vi "Path Get From Ini.vi"(11 "Ini Path":path caption="配置文件的路径") -> (0 "电压/流-1":cluster{"电压（V）":dbl, "电流（A）":dbl}, 1 "扫条码？":bool, 2 "图片路径":path, 3 "配置文件路径":path, 4 "打印？":bool caption="打印", 5 "取反":bool[](array[boolean]), 6 "MES路径":path, 7 "测试台类型":string, 8 "测连锡":bool)   [LabVIEW 2011]
uses:
  <vilib>/Utility/config.llb/Read Key (String).vi
  <vilib>/Utility/config.llb/Read Key (Boolean).vi
  <vilib>/Utility/config.llb/Read Key (Double).vi
  <vilib>/Utility/config.llb/Write Key (Double).vi
  <vilib>/Utility/config.llb/Write Key (Boolean).vi
  <vilib>/Utility/config.llb/NI_LVConfig.lvlib
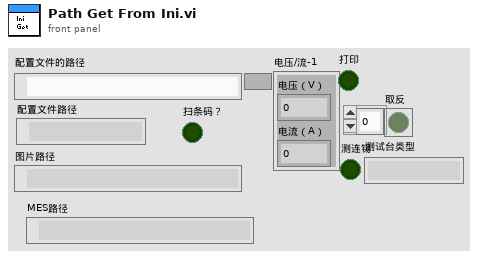
[diagram p1: front panel]
types:
  T1 = typedef "NI_LVConfig.lvlib/Config Data RefNum.ctl" = refnum<k1>
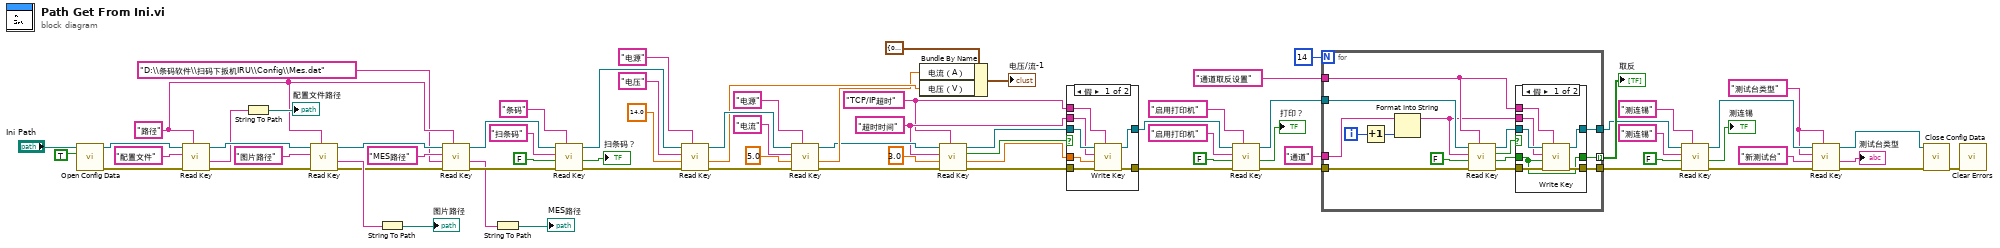
[diagram p0: block diagram]
diagram:
  w4 = "超时时间" ("key")
  w2 = "TCP/IP超时" ("section")
  w13 = "测试台类型" ("section")
  w35 = "路径" ("section")
  n1 = call <vilib>:"Open Config Data.vi"("create file if necessary (T)"=TRUE, "configuration file path"="Ini Path") -> ("error out"=w68:errorcluster, "refnum"=w74:T1)  [unwired: 7 in, 1 out]
  n2 = call-poly <vilib>:"Read Key.vi"("section"=w35, "error in (no error)"=w68, "key"="配置文件", "refnum"=w74) -> ("error out"=w67:errorcluster, "value"=w66:string, "refnum out"=w70:T1)  [unwired: 4 in, 1 out]
  n3 = String To Path(string=w66) -> (path=→"配置文件路径":path)
  n4 = call-poly <vilib>:"Read Key.vi"("section"=w35, "error in (no error)"=w67, "key"="图片路径", "refnum"=w70) -> ("error out"=w37:errorcluster, "value"=w65:string, "refnum out"=w39:T1)  [unwired: 4 in, 1 out]
  n5 = String To Path(string=w65) -> (path=→"图片路径":path)
  n6 = call-poly <vilib>:"Read Key.vi"("section"=w35, "error in (no error)"=w37, "default value"="D:\\条码软件\\扫码下扳机IRU\\Config\\Mes.dat", "key"="MES路径", "refnum"=w39) -> ("error out"=w36:errorcluster, "value"=w31:string, "refnum out"=w38:T1)  [unwired: 3 in, 1 out]
  n7 = String To Path(string=w31) -> (path=→"MES路径":path)
  n8 = call-poly <vilib>:"Read Key.vi"("section"="条码", "error in (no error)"=w36, "default value"=FALSE, "key"="扫条码", "refnum"=w38) -> ("error out"=w56:errorcluster, "value"=→"扫条码？":bool, "refnum out"=w57:T1)  [unwired: 3 in, 1 out]
  n9 = call-poly <vilib>:"Read Key.vi"("section"="电源", "error in (no error)"=w56, "default value"=14.0, "key"="电压", "refnum"=w57) -> ("error out"=w48:errorcluster, "value"=w45:dbl, "refnum out"=w49:T1)  [unwired: 3 in, 1 out]
  n10 = call-poly <vilib>:"Read Key.vi"("section"="电源", "error in (no error)"=w48, "default value"=5.0, "key"="电流", "refnum"=w49) -> ("error out"=w9:errorcluster, "value"=w44:dbl, "refnum out"=w10:T1)  [unwired: 3 in, 1 out]
  n11 = Bundle By Name(cluster=cluster{"电压（V）":dbl, "电流（A）":dbl} {"电压（V）"=0.0, "电流（A）"=0.0} ("电压/流-1 2"), "电流（A）"=w44, "电压（V）"=w45) -> (→"电压/流-1":cluster{"电压（V）":dbl, "电流（A）":dbl})
  n12 = call-poly <vilib>:"Read Key.vi"("section"=w2, "error in (no error)"=w9, "default value"=3.0, "key"=w4, "refnum"=w10) -> ("error out"=w7:errorcluster, "value"=w1:dbl, "found?"=w3:bool, "refnum out"=w8:T1)  [unwired: 3 in]
  n13 = case shown="假" w3 {
    tunnel: w8 -> [w81 w83]
    tunnel: w2 -> [w80 _]
    tunnel: w4 -> [w79 _]
    tunnel: w7 -> [w78 w82]
    tunnel: [w77 w82] -> w6
    tunnel: [w76 w83] -> w5
    tunnel: w1 -> [w75 _]
    frame False {
      n14 = call-poly <vilib>:"Write Key.vi"("section"=w80, "error in (no error)"=w78, "value"=w75, "key"=w79, "refnum"=w81) -> ("error out"=w77:errorcluster, "refnum out"=w76:T1)  [unwired: 4 in, 1 out]
    }
    frame True {
    }
  }
  n15 = call-poly <vilib>:"Read Key.vi"("section"="启用打印机", "error in (no error)"=w6, "default value"=FALSE, "key"="启用打印机", "refnum"=w5) -> ("error out"=w26:errorcluster, "value"=→"打印？":bool, "refnum out"=w27:T1)  [unwired: 3 in, 1 out]
  n16 = for {
    N: 14 -> [_]
    tunnel: w27 -> [w98]
    tunnel: w26 -> [w97]
    tunnel: "通道取反设置" ("名称或相对路径") -> [w90]
    tunnel: "通道" ("名称或相对路径") -> [w94]
    tunnel: [w87] -> w20
    tunnel: [w84] -> w21
    tunnel: [w86] -> w25 mode=indexing
    i -> [w96]
    n17 = Increment(x=w96) -> (x+1=w95:i32)
    n18 = Format Into String(initial string=w94, w95) -> (resulting string=w89:string)  [unwired: 2 in, 1 out]
    n19 = call-poly <vilib>:"Read Key.vi"("section"=w90, "error in (no error)"=w97, "default value"=FALSE, "key"=w89, "refnum"=w98) -> ("error out"=w88:errorcluster, "value"=w85:bool, "found?"=w92:bool, "refnum out"=w91:T1)  [unwired: 3 in]
    n20 = case shown="假" w92 {
      tunnel: w91 -> [w105 w108]
      tunnel: w90 -> [w104 _]
      tunnel: w89 -> [w103 _]
      tunnel: w88 -> [w102 w107]
      tunnel: [w101 w107] -> w87
      tunnel: [w100 w108] -> w84
      tunnel: [w99 w106] -> w86
      tunnel: w85 -> [w99 w106]
      frame False {
        n21 = call-poly <vilib>:"Write Key.vi"("section"=w104, "error in (no error)"=w102, "value"=w99, "key"=w103, "refnum"=w105) -> ("error out"=w101:errorcluster, "refnum out"=w100:T1)  [unwired: 4 in, 1 out]
      }
      frame True {
      }
    }
  }
  "取反" <- w25
  n22 = call-poly <vilib>:"Read Key.vi"("section"="测连锡", "error in (no error)"=w20, "default value"=FALSE, "key"="测连锡", "refnum"=w21) -> ("error out"=w16:errorcluster, "value"=→"测连锡":bool, "refnum out"=w18:T1)  [unwired: 3 in, 1 out]
  n23 = call-poly <vilib>:"Read Key.vi"("section"=w13, "error in (no error)"=w16, "default value"="新测试台" ("key"), "key"=w13, "refnum"=w18) -> ("error out"=w15:errorcluster, "value"=→"测试台类型":string, "refnum out"=w17:T1)  [unwired: 3 in, 1 out]
  n24 = call <vilib>:"Close Config Data.vi"("error in (no error)"=w15, "refnum"=w17) -> ("error out"=w62:errorcluster)  [unwired: 8 in, 1 out]
  n25 = call <vilib>:"Clear Errors.vi"("error in (no error)"=w62) -> ()  [unwired: 6 in, 1 out]
